vi "DAC_client.vi"(9 "manager":T1={"address"="localhost", "port"=7682, "password"=""}, 10 "update":bool, 11 "Channel":cluster{string, dbl}={"comp1", 1.0}) -> ()   [LabVIEW 2012]
uses:
  <userlib>/LabRAD/internal/Build Packet SubVIs/Build Packet by Name.vi
  <userlib>/LabRAD/internal/Simple Request SubVIs/Simple Request by Name.vi
panel:
  out "client ID":u32
  out "welcome message":string
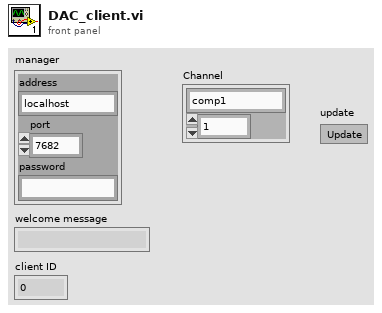
[diagram p1: front panel]
types:
  T1 = cluster{"address":string, "port":u16, "password":string}
  T2 = cluster{"Setting":cluster{"ID":u32, "Name":string}, "Type Tag":string, "Data":string}[]
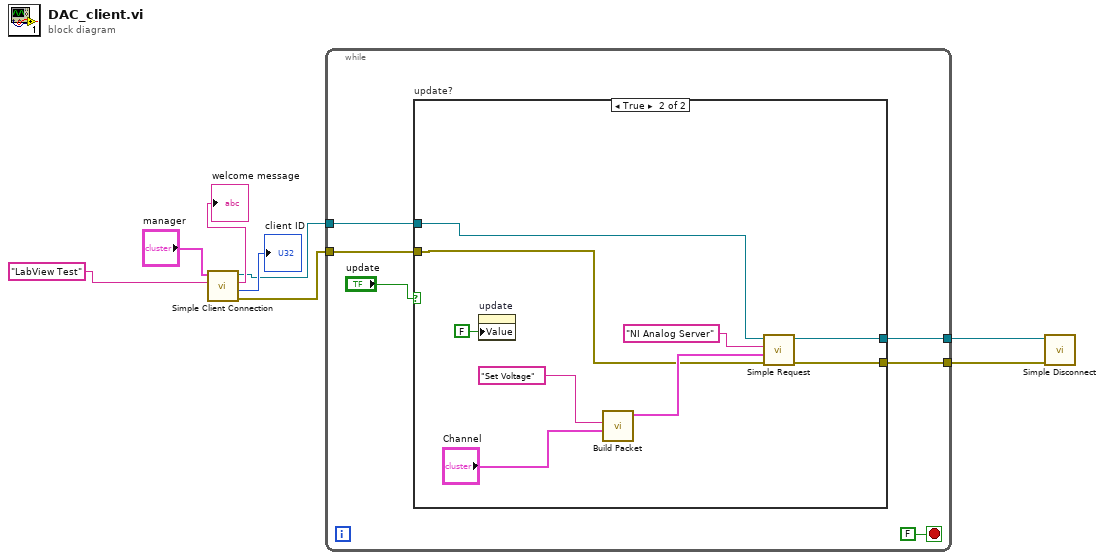
[diagram p0: block diagram]
diagram:
  n1 = call <userlib>:"Simple Client Connection.vi"("connection name (LabVIEW Client)"="LabView Test", "manager"="manager") -> ("error out"=w4:errorcluster, "client ID"=→"client ID":u32, "welcome message"=→"welcome message":string, "connection ID out"=w3:refnum<k5>)  [unwired: 2 in]
  n2 = while {
    tunnel: w4 -> [w12]
    tunnel: w3 -> [w11]
    tunnel: [w10] -> w2
    tunnel: [w9] -> w1
    stop <- FALSE stop-if-true
    n3 = case "update?" shown="True" "update" {
      tunnel: w12 -> [w15 w19]
      tunnel: w11 -> [w16 w20]
      tunnel: [w16 w18] -> w10
      tunnel: [w15 w17] -> w9
      frame False {
      }
      frame True {
        n4 = property on="update" class="Bool (strict)"("Value"=FALSE ("update")) -> ()  [unwired: 2 in, 2 out]
        n5 = call-poly <userlib>:"Build Packet.vi"("data (empty)"="Channel", "setting"="Set Voltage") -> ("appended records"=w23:T2)  [unwired: 6 in, 2 out]
        n6 = call-poly <userlib>:"Simple Request.vi"("error in (no error)"=w19, "records in (empty)"=w23, "target (Manager)"="NI Analog Server", "connection ID"=w20) -> ("error out"=w17:errorcluster, "connection ID out"=w18:refnum<k5>)  [unwired: 2 in, 2 out]
      }
    }
  }
  n7 = call <userlib>:"Simple Disconnect.vi"("error in (no error)"=w1, "connection ID"=w2) -> ()  [unwired: 5 in, 1 out]
